vi "Same Type.vi"() -> ()   [LabVIEW 2017, in "Transparent Assertions.Tests.lvlib" / "Assert Not Type.lvlib"]
uses:
  Assert Not Type.lvlib
  <vilib>/Utility/Data Type/Type Definitions/Data Type.ctl
  src/Transparent Assertions/Transparent Assertions.lvlib
  <vilib>/Utility/Data Type/NI_Data Type.lvlib
panel:
  out "error out":errorcluster
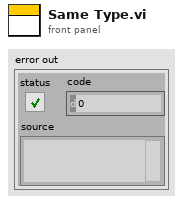
[diagram p1: front panel]
types:
  T1 = typedef "NI_Data Type.lvlib/Data Type.ctl" = enum8{"Invalid Type", "Void", "I8", "I16", "I32", "I64", "U8", "U16", "U32", "U64", "Single Float", "Double Float", "Extended Float", "Single Complex", "Double Complex", "Extended Complex", "Enum U8", "Enum U16", "Enum U32", "Enum U64", "Single Float With Unit", "Double Float With Unit", "Extended Float With Unit", "Single Complex with Unit", "Double Complex with Unit", "Extended Complex with Unit", "Boolean", "String", "Path", "Picture", "Tag", "Array", "Cluster", "Variant", "LV Variant", "Waveform", "Timestamp", "Digital Waveform", "Digital Data", "ExpressData", "Refnum", "External Data", "VI", "Poly VI", "LabVIEW Class Instance", "Fixed Point"}
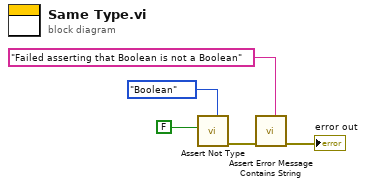
[diagram p0: block diagram]
diagram:
  n1 = call "Assert Not Type.vi"("Type"=Data_Type."Boolean", "Actual"=FALSE) -> ("error out"=w4:errorcluster)  [unwired: 9 in]
  n2 = call "Assert Error Message Contains String.vi"("Expected"="Failed asserting that Boolean is not a Boolean", "error in (no error)"=w4) -> ("error out"=→"error out":errorcluster)  [unwired: 9 in]
